vi "ToString.vi"(8 "error in (no error)":errorcluster, 11 "Constraint in":refnum<class "Constraint.lvclass">) -> (0 "error out":errorcluster, 2 "String":string, 3 "Constraint out":refnum<class "Constraint.lvclass">)   [LabVIEW 2017, in "Transparent Assertions.lvlib" / "Constraint.lvclass"]
doc: "Returns a string representation of the object."
uses:
  Constraint.lvclass
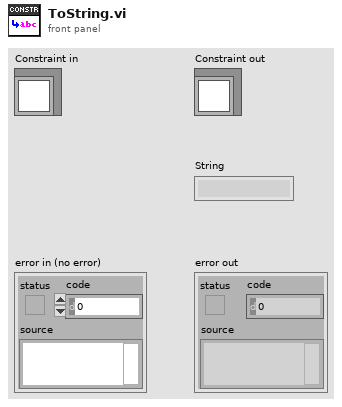
[diagram p1: front panel]
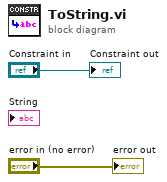
[diagram p0: block diagram]
diagram:
  "error out" <- "error in (no error)"
  "Constraint out" <- "Constraint in"
